vi "Result_Test.vi"(8 "error in (no error)":errorcluster caption="entrée d'erreur (pas d'erreur)", 11 "Flash_Jlink en entrée":refnum<class "Flash_P2056.lvclass">) -> (0 "error out":errorcluster caption="sortie d'erreur", 3 "Flash_Jlink en sortie":refnum<class "Flash_P2056.lvclass">)   [LabVIEW 2020, in "Library Test.lvlib" / "Flash_P2056.lvclass"]
uses:
  Flash_P2056.lvclass
  C:/Users/ngarcin/OneDrive - Altyor/Standard TB/Class/Test/Test (Default)/Test (Default).lvclass
  Test_Without_Instr/Test_Without_Inst.lvclass
  Flash_P2056.lvclass/Flash_P2056.ctl
panel:
  out "standard output":string caption="sortie standard"
  out "Ok":bool
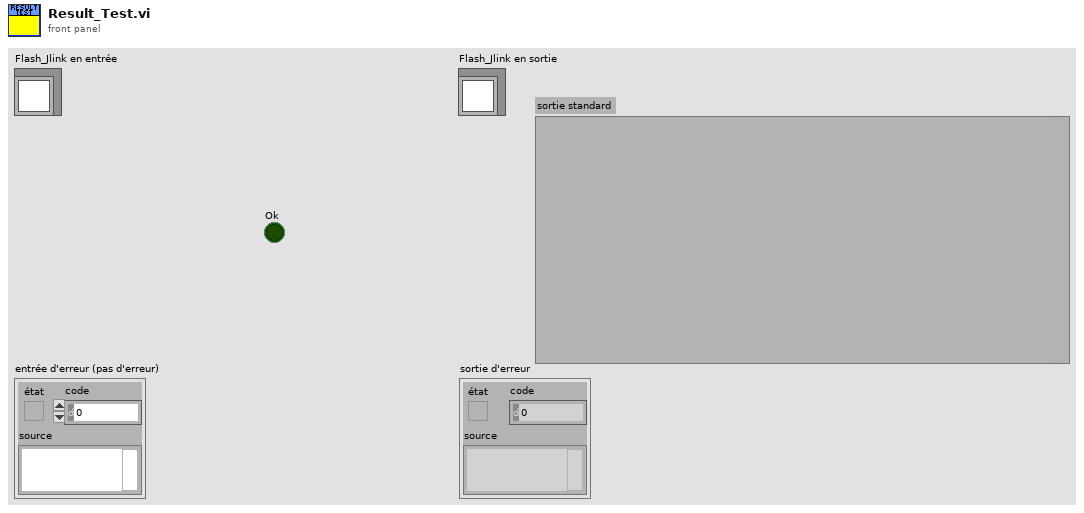
[diagram p1: front panel]
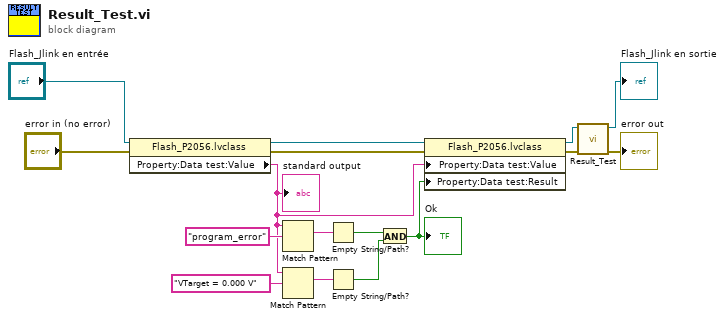
[diagram p0: block diagram]
diagram:
  n1 = property class="Flash_P2056.lvclass"(reference="Flash_Jlink en entrée", error in="error in (no error)") -> (reference out=w9:refnum<class "Flash_P2056.lvclass">, error out=w11:errorcluster, "Property:Data test:Value"=w1:string)
  "standard output" <- w1
  n2 = Match Pattern(string=w1, regular expression="program_error" ("expression régulière")) -> (match substring=w8:string)  [unwired: 1 in, 3 out]
  n3 = Match Pattern(string=w1, regular expression="VTarget = 0.000 V" ("expression régulière")) -> (match substring=w5:string)  [unwired: 1 in, 3 out]
  n4 = Empty String/Path?(string/path=w8) -> (empty?=w4:bool)
  n5 = Empty String/Path?(string/path=w5) -> (empty?=w3:bool)
  n6 = And(x=w4, y=w3) -> (x .and. y?=w2:bool)
  "Ok" <- w2
  n7 = property class="Flash_P2056.lvclass"(reference=w9, error in=w11, "Property:Data test:Value"=w1, "Property:Data test:Result"=w2) -> (reference out=w13:refnum<class "Flash_P2056.lvclass">, error out=w16:errorcluster)
  n8 = call-parent "Result_Test.vi"("error in (no error)"=w16, "Test_Without_Inst en entrée"=w13) -> ("error out"=→"error out":errorcluster, "Test_Without_Inst en sortie"=→"Flash_Jlink en sortie":refnum<class "Flash_P2056.lvclass">)  [unwired: 8 in]
